vi "Get Class and Ancestor Methods from Class Library.vi"(0 "Class Library Ref":refnum<vi>, 3 "error in":errorcluster) -> (4 "Access Scopes":T1(array[ring]), 5 "Wire Pens":T2(array[cluster]), 6 "dup Ref":refnum<vi>, 7 "Method Names":string[](array[string]), 8 "Method VIs":refnum<vi>[](array[refnum]), 9 "error out":errorcluster)   [LabVIEW 2025, in "XNode Support.lvlib"]
uses:
  XNode Support.lvlib
  <vilib>/regexp/Match Regular Expression.xnode
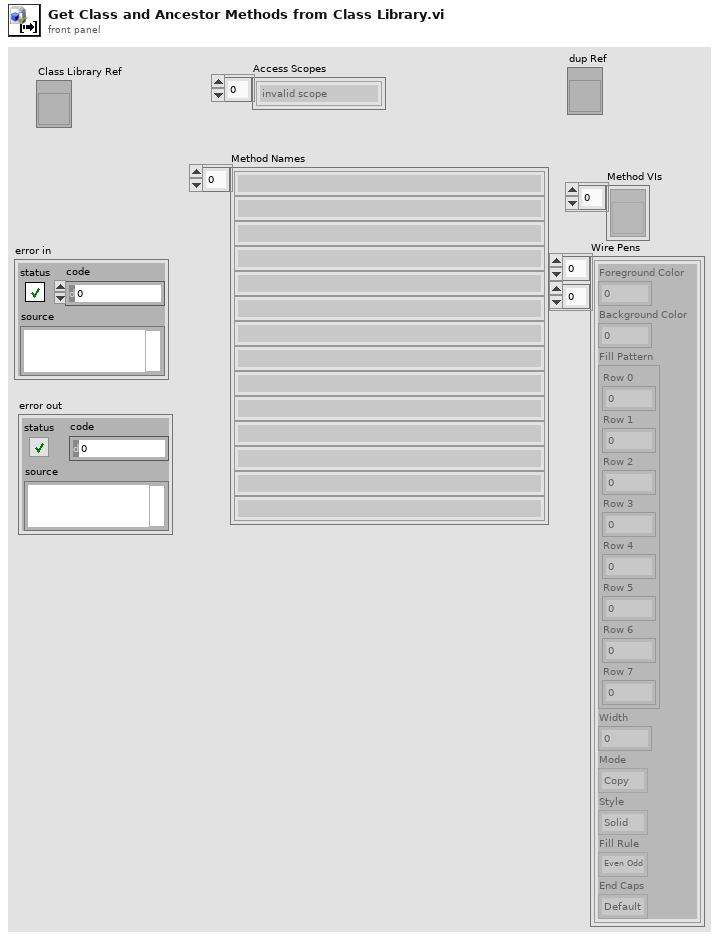
[diagram p1: front panel]
types:
  T1 = enum32{"invalid scope", "public", "private", "protected", "community"}[]
  T2 = cluster{"Foreground Color":u32, "Background Color":u32, "Fill Pattern":cluster{"Row 0":u8, "Row 1":u8, "Row 2":u8, "Row 3":u8, "Row 4":u8, "Row 5":u8, "Row 6":u8, "Row 7":u8}, "Width":i16, "Mode":enum16{"Copy", "Or", "Exclusive Or", "Bit Clear", "Not Copy", "Not Or", "Nor Exclusive Or", "Not Bit Clear"}, "Style":enum32{"Solid", "Dash", "Dot", "Dash Dot", "Dash Dot Dot"}, "Fill Rule":enum32{"Even Odd", "Winding"}, "End Caps":enum32{"Default", "Flat"}}[][]
  T3 = enum32{"invalid scope", "public", "private", "protected", "community"}
  T4 = enum32{"invalid VI type", "Standard VI", "Control VI", "Global VI", "Polymorphic VI", "Configuration VI", "SubSystem", "Facade VI", "Method VI", "Statechart Diagram VI"}
  T5 = cluster{"Foreground Color":u32, "Background Color":u32, "Fill Pattern":cluster{"Row 0":u8, "Row 1":u8, "Row 2":u8, "Row 3":u8, "Row 4":u8, "Row 5":u8, "Row 6":u8, "Row 7":u8}, "Width":i16, "Mode":enum16{"Copy", "Or", "Exclusive Or", "Bit Clear", "Not Copy", "Not Or", "Nor Exclusive Or", "Not Bit Clear"}, "Style":enum32{"Solid", "Dash", "Dot", "Dash Dot", "Dash Dot Dot"}, "Fill Rule":enum32{"Even Odd", "Winding"}, "End Caps":enum32{"Default", "Flat"}}[]
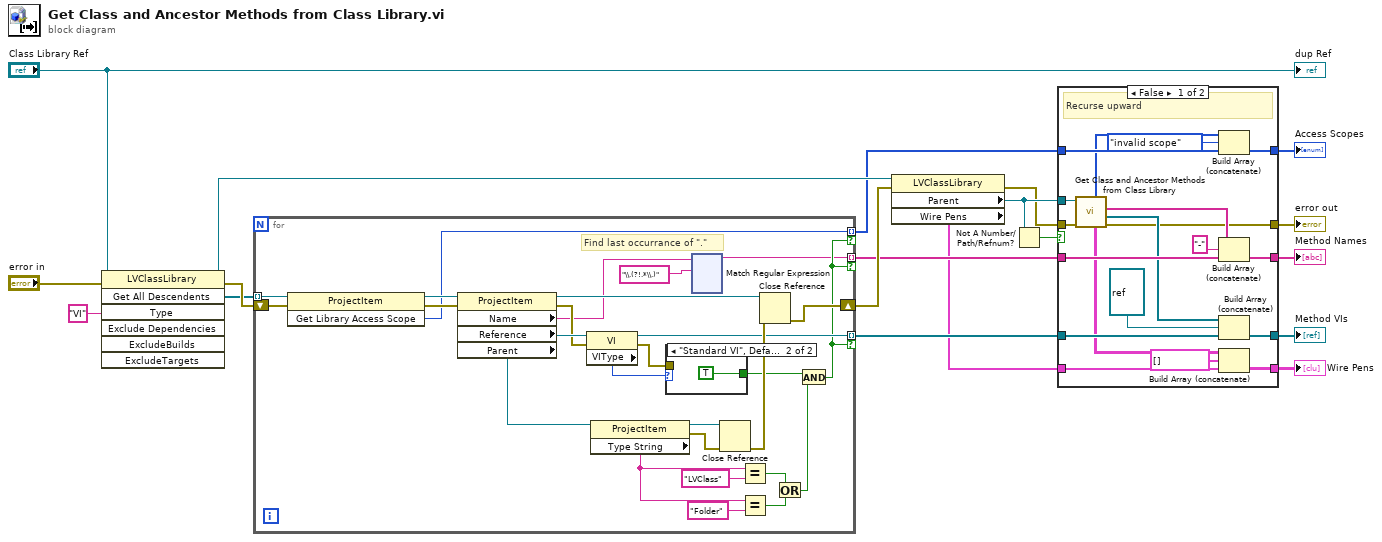
[diagram p0: block diagram]
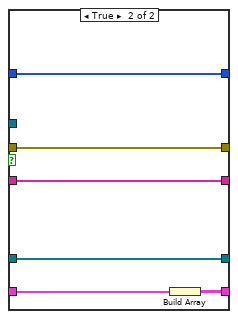
[diagram p3: hidden frame]
diagram:
  n1 = invoke class="LVClassLibrary" method="Get All Descendents"(reference="Class Library Ref", error in="error in", "Type"="VI") -> (reference out=w16:refnum<vi>, error out=w18:errorcluster, "All Descendents"=w17:refnum<vi>[])  [unwired: 4 in, 4 out]
  n2 = for {
    tunnel: w17 -> [w25] mode=indexing
    tunnel: [w38] -> w7 mode=indexing if=w23
    tunnel: [w20] -> w11 mode=indexing if=w23
    shift-right: [w40] -> w19
    shift-left: w18 -> [w27]
    tunnel: [w24] -> w6 mode=indexing if=w23
    # "Find last occurrance of \".\""
    n3 = invoke class="ProjectItem" method="Get Library Access Scope"(reference=w25, error in=w27) -> (reference out=w28:refnum<vi>, error out=w26:errorcluster, "Get Library Access Scope"=w24:T3)  [unwired: 1 in]
    n4 = property class="ProjectItem"(reference=w28, error in=w26) -> (reference out=w42:refnum<vi>, error out=w37:errorcluster, "Name"=w21:string, "Reference"=w39:refnum<vi>, "Parent"=w46:refnum<vi>)
    n5 = property class="VI"(reference=w39, error in=w37) -> (reference out=w38:refnum<vi>, error out=w34:errorcluster, "VIType"=w36:T4)
    n6 = property class="ProjectItem"(reference=w46) -> (reference out=w44:refnum<vi>, error out=w43:errorcluster, "Type String"=w32:string)  [unwired: 1 in]
    n7 = case shown="\"Standard VI\", Default" w36 {
      tunnel: [_ TRUE] -> w35
      tunnel: w34 -> [_ _]
      frame "invalid VI type", "Control VI", "Global VI" {
      }
      frame "Standard VI", Default {
      }
    }
    n8 = xnode "Match Regular Expression"("input string"=w21, "regular expression"="\\.(?!.*\\.)") -> ("before match"=w20:string)  [unwired: 4 in, 4 out]
    n9 = Close Reference(reference=w44, error in (no error)=w43) -> (error out=w41:errorcluster)
    n10 = Equal?(x=w32, y="LVClass") -> (x = y?=w30:bool)
    n11 = Equal?(x=w32, y="Folder") -> (x = y?=w31:bool)
    n12 = Close Reference(reference=w42, error in (no error)=w41) -> (error out=w40:errorcluster)
    n13 = Or(x=w30, y=w31) -> (x .or. y?=w29:bool)
    n14 = And(x=w35, y=w29) -> (x .and. y?=w23:bool)
  }
  n15 = property class="LVClassLibrary"(reference=w16, error in=w19) -> (error out=w8:errorcluster, "Parent"=w12:refnum<vi>, "Wire Pens"=w1:T5)  [unwired: 1 out]
  n16 = Not A Number/Path/Refnum?(number/path/refnum=w12) -> (NaN/Path/Refnum?=w13:bool)
  n17 = case shown="False" w13 {
    tunnel: w12 -> [w166 _]
    tunnel: w11 -> [w183 w189]
    tunnel: [w182 w189] -> w10
    tunnel: w8 -> [w179 w186]
    tunnel: w7 -> [w178 w188]
    tunnel: w6 -> [w174 w187]
    tunnel: [w177 w188] -> w5
    tunnel: [w173 w187] -> w4
    tunnel: [w170 w186] -> w3
    tunnel: w1 -> [w168 w185]
    tunnel: [w167 w184] -> w2
    frame False {
      # "Recurse upward"
      n18 = call "Get Class and Ancestor Methods from Class Library.vi"("Class Library Ref"=w166, "error in"=w179) -> ("Access Scopes"=w171:T1, "Wire Pens"=w169:T2, "Method Names"=w181:string[], "Method VIs"=w176:refnum<vi>[], "error out"=w170:errorcluster)  [unwired: 2 in, 1 out]
      n19 = Build Array (concatenate)(w171, T3."invalid scope" ("array"), w174) -> (w173:T1)
      n20 = Build Array (concatenate)(w181, "-", w183) -> (w182:string[])
      n21 = Build Array (concatenate)(w176, refnum<vi> refnum ("Reference"), w178) -> (w177:refnum<vi>[])
      n22 = Build Array (concatenate)(w169, T5 [] ("array"), w168) -> (w167:T2)
    }
    frame True {
      n23 = Build Array(w185) -> (w184:T2)
    }
  }
  "Method Names" <- w10
  "Method VIs" <- w5
  "error out" <- w3
  "Wire Pens" <- w2
  "Access Scopes" <- w4
  "dup Ref" <- "Class Library Ref"
